vi "SENS_FREQ_SPAN.vi"(0 "VISA IN":refnum<visa-resource-name>, 1 "Frq. Span":dbl, 5 "error in":errorcluster, 7 "Channel":i32) -> (14 "VISA Out":refnum<visa-resource-name>, 19 "error out":errorcluster)   [LabVIEW 2018, in "PNA-X.lvlib"]
doc: "SENSe<cnum>:FREQuency:SPAN <num> \n(Read-Write) Sets the frequency span of the analyzer. \nParameters \n<cnum> Any existing channel number. If unspecified, value is set to 1 \n<num> Frequency span. Choose any number between: \n0 (minimum) and the maximum frequency span of the analyzer. \nUnits are Hz \nSee Note \nExamples SENS:FREQ:SPAN 1000000 \nsense2:frequency:span max \nQuery Syntax SENSe<cnum>:FREQuency:SPAN? \nReturn Type Numeric \nDefault Maximum frequency span of the analyzer"
uses:
  PNA-X.lvlib
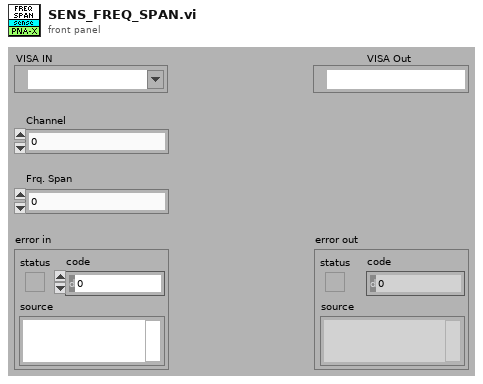
[diagram p1: front panel]
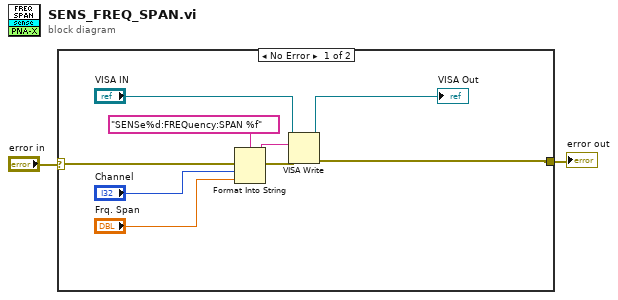
[diagram p0: block diagram]
diagram:
  n1 = case shown="No Error" "error in" {
    selector: "error in" -> [w11 w12]
    tunnel: [w6 w12] -> w1
    frame No Error {
      n2 = Format Into String(format string="SENSe%d:FREQuency:SPAN %f" ("Cmdline"), error in=w11, "Channel", "Frq. Span") -> (resulting string=w9:string, error out=w10:errorcluster)  [unwired: 1 in]
      n3 = VISA Write(VISA resource name="VISA IN", write buffer=w9, error in (no error)=w10) -> (VISA resource name out=→"VISA Out":refnum<visa-resource-name>, error out=w6:errorcluster)  [unwired: 1 out]
    }
    frame Error {
    }
  }
  "error out" <- w1
